vi "CleanUp.vi"(0 "object in":refnum<class "ABCPassPlay.lvclass">, 5 "error in (no error)":errorcluster) -> (14 "object out":refnum<class "ABCPassPlay.lvclass">, 19 "error out":errorcluster)   [LabVIEW 2021, in "ABCPassPlay.lvclass"]
uses:
  ABCPassPlay.lvclass
  Play_class/Play.lvclass
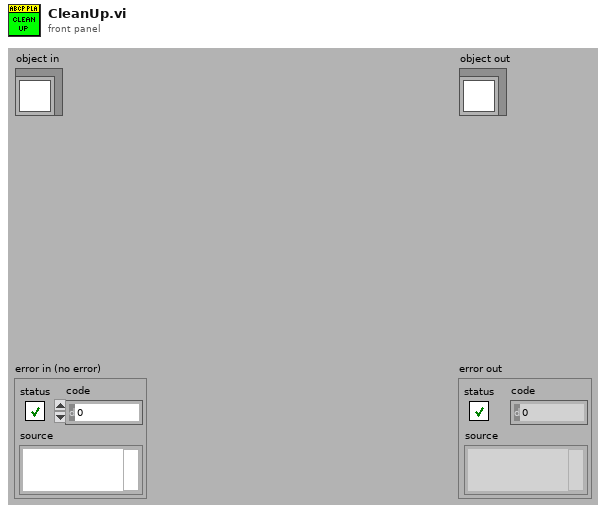
[diagram p1: front panel]
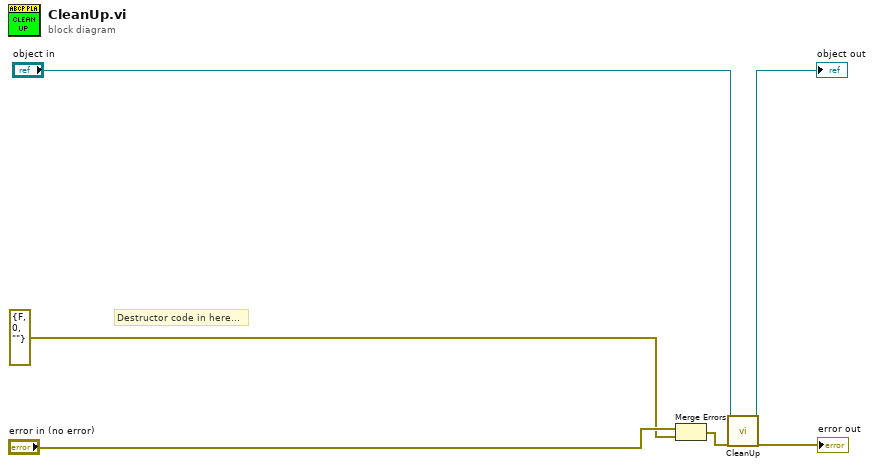
[diagram p0: block diagram]
diagram:
  # "Destructor code in here..."
  n1 = Merge Errors("error in (no error)", errorcluster {"status"=FALSE, "code"=0, "source"=""} ("error in (no error)")) -> (w4:errorcluster)
  n2 = call-parent "CleanUp.vi"("object in"="object in", "error in (no error)"=w4) -> ("object out"=→"object out":refnum<class "ABCPassPlay.lvclass">, "error out"=→"error out":errorcluster)  [unwired: 16 in]
